vi "Test Component A Does Something.vi"(11 "Test Case In":refnum<class "Component B Test.lvclass">) -> (0 "error out":errorcluster, 3 "Test Case Out":refnum<class "Component B Test.lvclass">)   [LabVIEW 2020, in "Component B Test Suite.lvlib" / "Component B Test.lvclass"]
uses:
  Component B Test.lvclass
  C:/git/astemes-lunit/source/LUnit Test Case.lvclass
  LUnit Test Case.lvclass/LUnit Test Case.ctl
  c4973807-a8e3-4cb3-961c-4b1521e4df90.vi
  Core/LUnit Test Case/Private/Append Pass Result.vi
  Core/LUnit Test Case/Private/Append Fail Result.vi
  c4973807-a8e3-4cb3-961c-4b1521e4df90.vi/9c5d11cd-9439-4240-a1ee-d9baace9c924.vi
  Core/LUnit Test Case/Private/Run In UI.vi
  <vilib>/Utility/error.llb/Clear Errors.vi
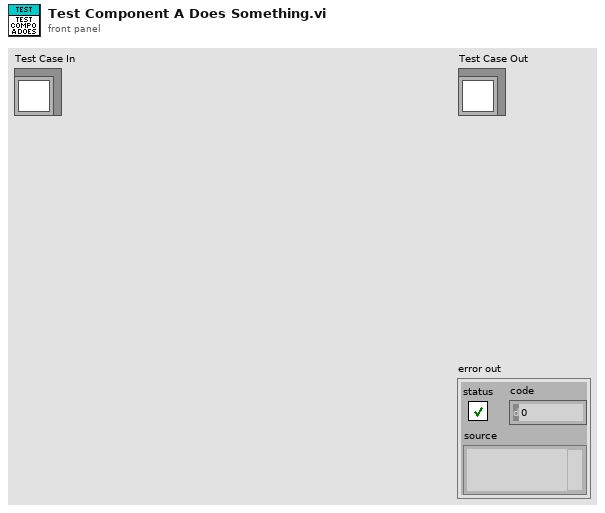
[diagram p1: front panel]
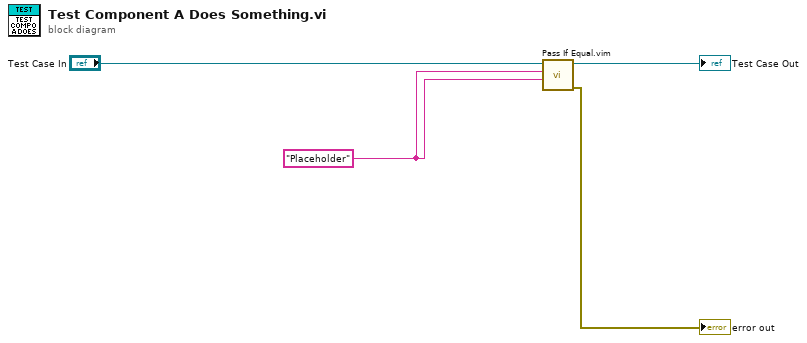
[diagram p0: block diagram]
diagram:
  w1 = "Placeholder"
  n1 = call "Pass If Equal.vim"("Actual"=w1, "Expected"=w1, "LUnit Test Case In"="Test Case In") -> ("error out"=→"error out":errorcluster, "LUnit Test Case Out"=→"Test Case Out":refnum<class "Component B Test.lvclass">)  [unwired: 7 in]
